vi "ClearXYZTheta Go.vi"(8 "error in (no error)":errorcluster, 10 "XYZTheta In":dbl[](array[numeric]), 11 "Gantry In":refnum<k24>) -> (0 "error out":errorcluster, 2 "XYZTheta Out":dbl[](array[numeric]), 3 "Gantry Out":refnum<k24>)   [LabVIEW 2021, in "Motion.lvclass"]
uses:
  Motion.lvclass
  C:/Program Files (x86)/Aerotech/A3200/LabVIEW/2010/Bin/Aerotech.A3200.dll
  Program Files (x86)/Aerotech/A3200/LabVIEW/2010/Bin/Aerotech.A3200.dll
  A3200/A3200.lvclass
  Drivers/Aerotech A3200/Aerotech.lvlib
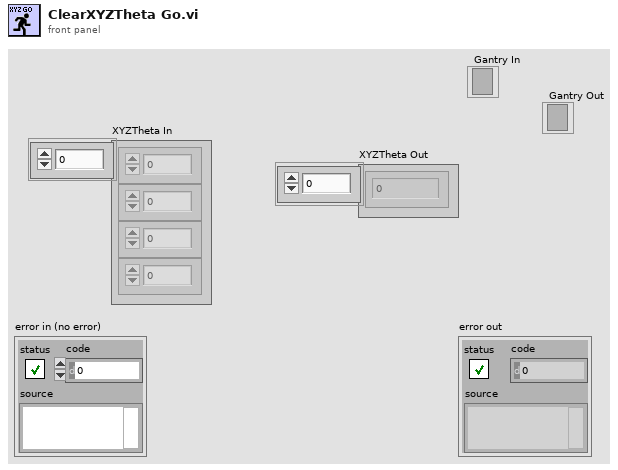
[diagram p1: front panel]
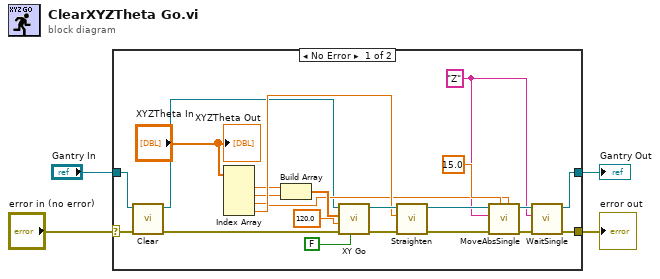
[diagram p0: block diagram]
diagram:
  n1 = case shown="No Error" "error in (no error)" {
    selector: "error in (no error)" -> [w9 w28]
    tunnel: [w5 w28] -> w3
    tunnel: "Gantry In" -> [w11 w27]
    tunnel: [w13 w27] -> w1
    frame No Error {
      w12 = "Z" ("axis name")
      n2 = call "Clear.vi"("error in (no error)"=w9, "Gantry In"=w11) -> ("error out"=w8:errorcluster, "Gantry Out"=w10:refnum<k24>)  [unwired: 8 in]
      n3 = Index Array(array="XYZTheta In") -> (element #1=w21:dbl, element #2=w20:dbl, element #3=w16:dbl, element #4=w23:dbl)  [unwired: 4 in]
      n4 = Build Array(w21, w20) -> (w22:dbl[])
      n5 = call "XY Go.vi"("return immediately"=FALSE, "error in (no error)"=w8, "Speed"=120.0, "XY In"=w22, "Gantry In"=w10) -> ("error out"=w19:errorcluster, "Gantry Out"=w24:refnum<k24>)  [unwired: 4 in, 1 out]
      n6 = call "Straighten.vi"("error in (no error)"=w19, "Angle (rad)"=w23, "Gantry In"=w24) -> ("error out"=w15:errorcluster, "Gantry Out"=w18:refnum<k24>)  [unwired: 7 in]
      n7 = call "MoveAbsSingle.vi"("position"=w16, "speed"=15.0, "error in (no error)"=w15, "axis name"=w12, "controller in"=w18) -> ("error out"=w6:errorcluster, "controller out"=w14:refnum<k24>)  [unwired: 5 in]
      n8 = call "WaitSingle.vi"("error in (no error)"=w6, "axis name"=w12, "controller in"=w14) -> ("error out"=w5:errorcluster, "controller out"=w13:refnum<k24>)  [unwired: 6 in, 1 out]
      "XYZTheta Out" <- "XYZTheta In"
    }
    frame Error {
    }
  }
  "error out" <- w3
  "Gantry Out" <- w1
